vi "UI_Size.vi"(1 "引用":refnum<vi>, 2 "确定按钮":bool, 3 "宽":i16=564, 4 "高":i16=459) -> ()   [LabVIEW 2016]
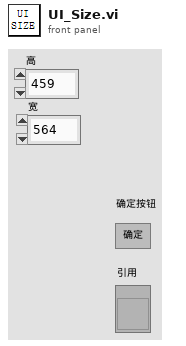
[diagram p1: front panel]
types:
  T1 = typedef "LVRectTypeDef.ctl" = cluster{"Left":i16, "Top":i16, "Right":i16, "Bottom":i16}
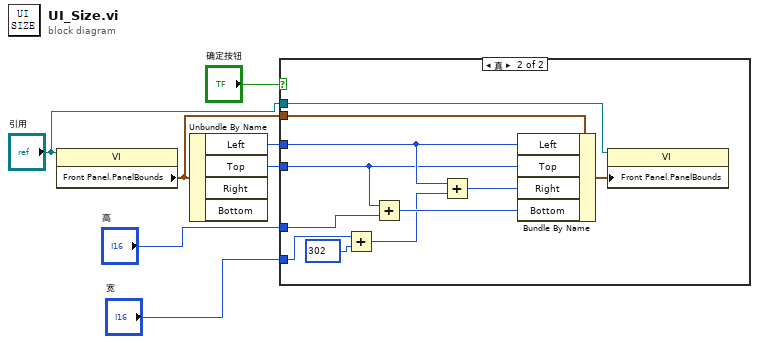
[diagram p0: block diagram]
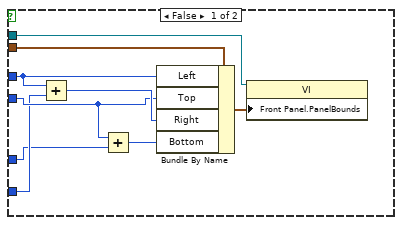
[diagram p2: hidden frame]
diagram:
  n1 = property class="VI"(reference="引用") -> ("Front Panel.PanelBounds"=w7:T1)  [unwired: 1 in, 2 out]
  n2 = Unbundle By Name(w7) -> ("Left"=w6:i16, "Top"=w5:i16)  [unwired: 2 out]
  n3 = case shown="真" "确定按钮" {
    tunnel: w7 -> [w15 w23]
    tunnel: w6 -> [w13 w24]
    tunnel: w5 -> [w12 w22]
    tunnel: "引用" -> [w10 w21]
    tunnel: "宽" -> [w9 w20]
    tunnel: "高" -> [w8 w17]
    frame False {
      n4 = Add(x=w13, y=w9) -> (x+y=w14:i16)
      n5 = Add(x=w12, y=w8) -> (x+y=w11:i16)
      n6 = Bundle By Name(cluster=w15, "Left"=w13, "Top"=w12, "Right"=w14, "Bottom"=w11) -> (w16:T1)
      n7 = property class="VI"(reference=w10, "Front Panel.PanelBounds"=w16) -> ()  [unwired: 1 in, 2 out]
    }
    frame True {
      n8 = Add(x=w20, y=i16 302) -> (x+y=w18:i16)
      n9 = Add(x=w22, y=w17) -> (x+y=w25:i16)
      n10 = Add(x=w24, y=w18) -> (x+y=w26:i16)
      n11 = Bundle By Name(cluster=w23, "Left"=w24, "Top"=w22, "Right"=w26, "Bottom"=w25) -> (w27:T1)
      n12 = property class="VI"(reference=w21, "Front Panel.PanelBounds"=w27) -> ()  [unwired: 1 in, 2 out]
    }
  }
